vi "仪器面板_时间判断子VI.vi"(2 "步长":dbl, 3 "起始时间":dbl, 4 "时间":dbl) -> (0 "x = y?":bool, 1 "连接的字符串":string)   [LabVIEW 2014]
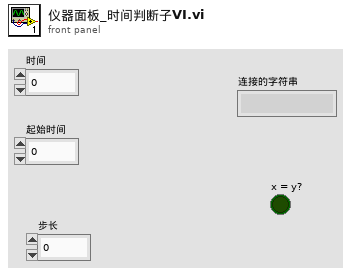
[diagram p1: front panel]
types:
  T1 = typedef "LVDateTimeRec.ctl" = cluster{"秒数的小数部分":dbl, "秒":i32, "分":i32, "时":i32, "日":i32, "月":i32, "年":i32, "天数（周）":i32, "天数（年）":i32, "DST":i32}
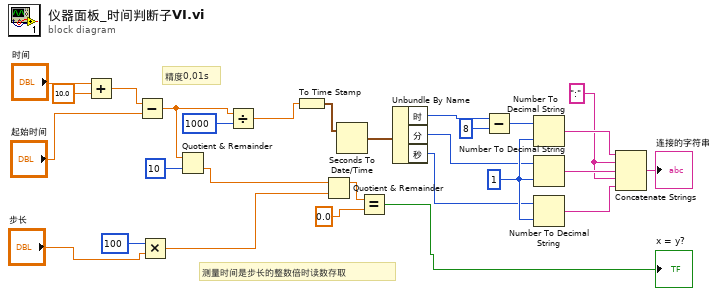
[diagram p0: block diagram]
diagram:
  w20 = i16 1 ("宽度(-)")
  w16 = ":" ("字符串")
  # "测量时间是步长的整数倍时读数存取"
  # "精度0,01s"
  n1 = Add(x="时间", y=10.0) -> (x+y=w26:dbl)
  n2 = Subtract(x=w26, y="起始时间") -> (x-y=w6:dbl)
  n3 = Multiply(x=100, y="步长") -> (x*y=w2:dbl)
  n4 = Quotient & Remainder(x=w6, y=u32 10) -> (floor(x/y)=w5:dbl)  [unwired: 1 out]
  n5 = Divide(x=w6, y=u32 1000) -> (x/y=w9:dbl)
  n6 = To Time Stamp(1:w9) -> (0:w19:timestamp)
  n7 = Quotient & Remainder(x=w5, y=w2) -> (x-y*floor(x/y)=w23:dbl)  [unwired: 1 out]
  n8 = Seconds To Date/Time(time stamp (now)=w19) -> (date time rec=w10:T1)  [unwired: 1 in]
  n9 = Equal?(x=w23, y=0.0) -> (x = y?=→"x = y?":bool)
  n10 = Unbundle By Name(w10) -> ("时"=w11:i32, "分"=w14:i32, "秒"=w15:i32)
  n11 = Subtract(x=w11, y=8) -> (x-y=w13:i32)
  n12 = Number To Decimal String(number=w13, width (-)=w20) -> (decimal integer string=w17:string)
  n13 = Number To Decimal String(number=w14, width (-)=w20) -> (decimal integer string=w18:string)
  n14 = Number To Decimal String(number=w15, width (-)=w20) -> (decimal integer string=w21:string)
  n15 = Concatenate Strings(w17, w16, w18, w16, w21) -> (→"连接的字符串":string)
